vi "GetEncScanSpan.vi"(8 "错误输入（无错误）":errorcluster, 11 "编码器序号":i32) -> (0 "错误输出":errorcluster, 3 "返回值":u8)   [LabVIEW 2014]
uses:
  X86Dll/ZXUTConfigMgr.dll
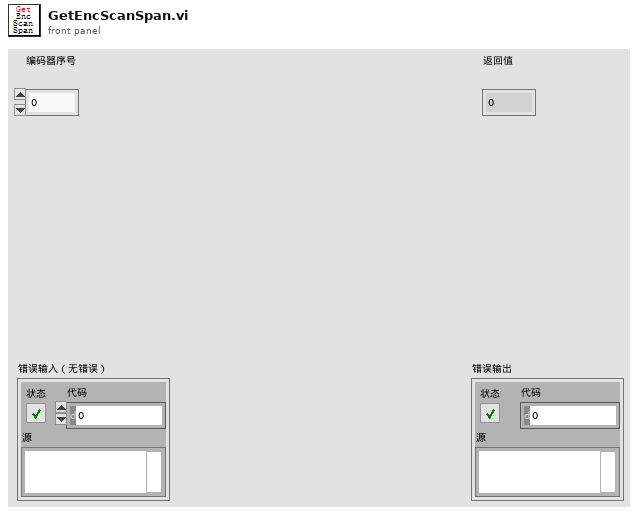
[diagram p1: front panel]
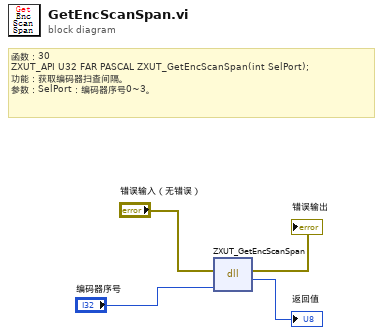
[diagram p0: block diagram]
diagram:
  # "函数：30\nZXUT_API U32\tFAR PASCAL ZXUT_GetEncScanSpan(int SelPort);\n功能：获取编码器扫查间隔。\n参数：SelPort：编码器序号0~3。"
  n1 = dll-call lib="D:/Software/Utrasonic on-line monitoring/X86Dll/ZXUTConfigMgr.dll" fn="ZXUT_GetEncScanSpan"(error in="错误输入（无错误）", "SelPort"="编码器序号") -> (error out=→"错误输出":errorcluster, "返回值"=→"返回值":u32)  [unwired: 3 in, 1 out]
